vi "TagSync.vi"() -> ()   [LabVIEW 2015]
uses:
  <vilib>/Utility/error.llb/DialogType.ctl
  <resource>/objmgr/daqmx.rc
  <vilib>/DAQmx/configure/timing.llb/DAQmx Timing (Sample Clock).vi
  <vilib>/DAQmx/create/channels.llb/DAQmx Create Channel (DO-Digital Output).vi
  <vilib>/DAQmx/write.llb/DAQmx Write (Digital Wfm 1Chan NSamp).vi
panel:
  in  "Sync Tagging":T1(tab)
  out "Minimum tagging period (pws)":u32=87
  out "Total tag data length (pws)":i32=86
  in  "Tagging Period (pws)":u32=155
  in  "Calculate recommended tag settings":bool
  in  "Validate tag settings":bool
  in  "Tag Marker Duration (pws)":i32=10
  in  "Requested Pulse Width (ms)":dbl=10.0
  out "Actual pulse width (ms)":dbl=-1.0
  in  "Sync Tag Output Line":tag
  in  "Sample Clock Source":tag
  out "Current tag period":digitalwaveform(graph)
  out "Current tag ID":u32=1
  in  "Enable monitoring":bool
  in  "Min extra tag separation (pws)":u32=1
  in  "Minimum tags per file":u32=3
  in  "Minimum samples per pulse":dbl=10.0 format="%#_13g"
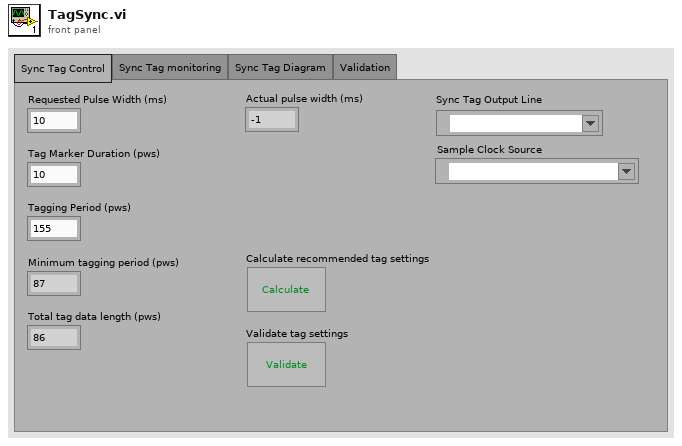
[diagram p1: front panel]
types:
  T1 = enum32{"Sync Tag Control", "Sync Tag monitoring", "Sync Tag Diagram", "Validation"}
  T2 = typedef "DialogType.ctl" = u16
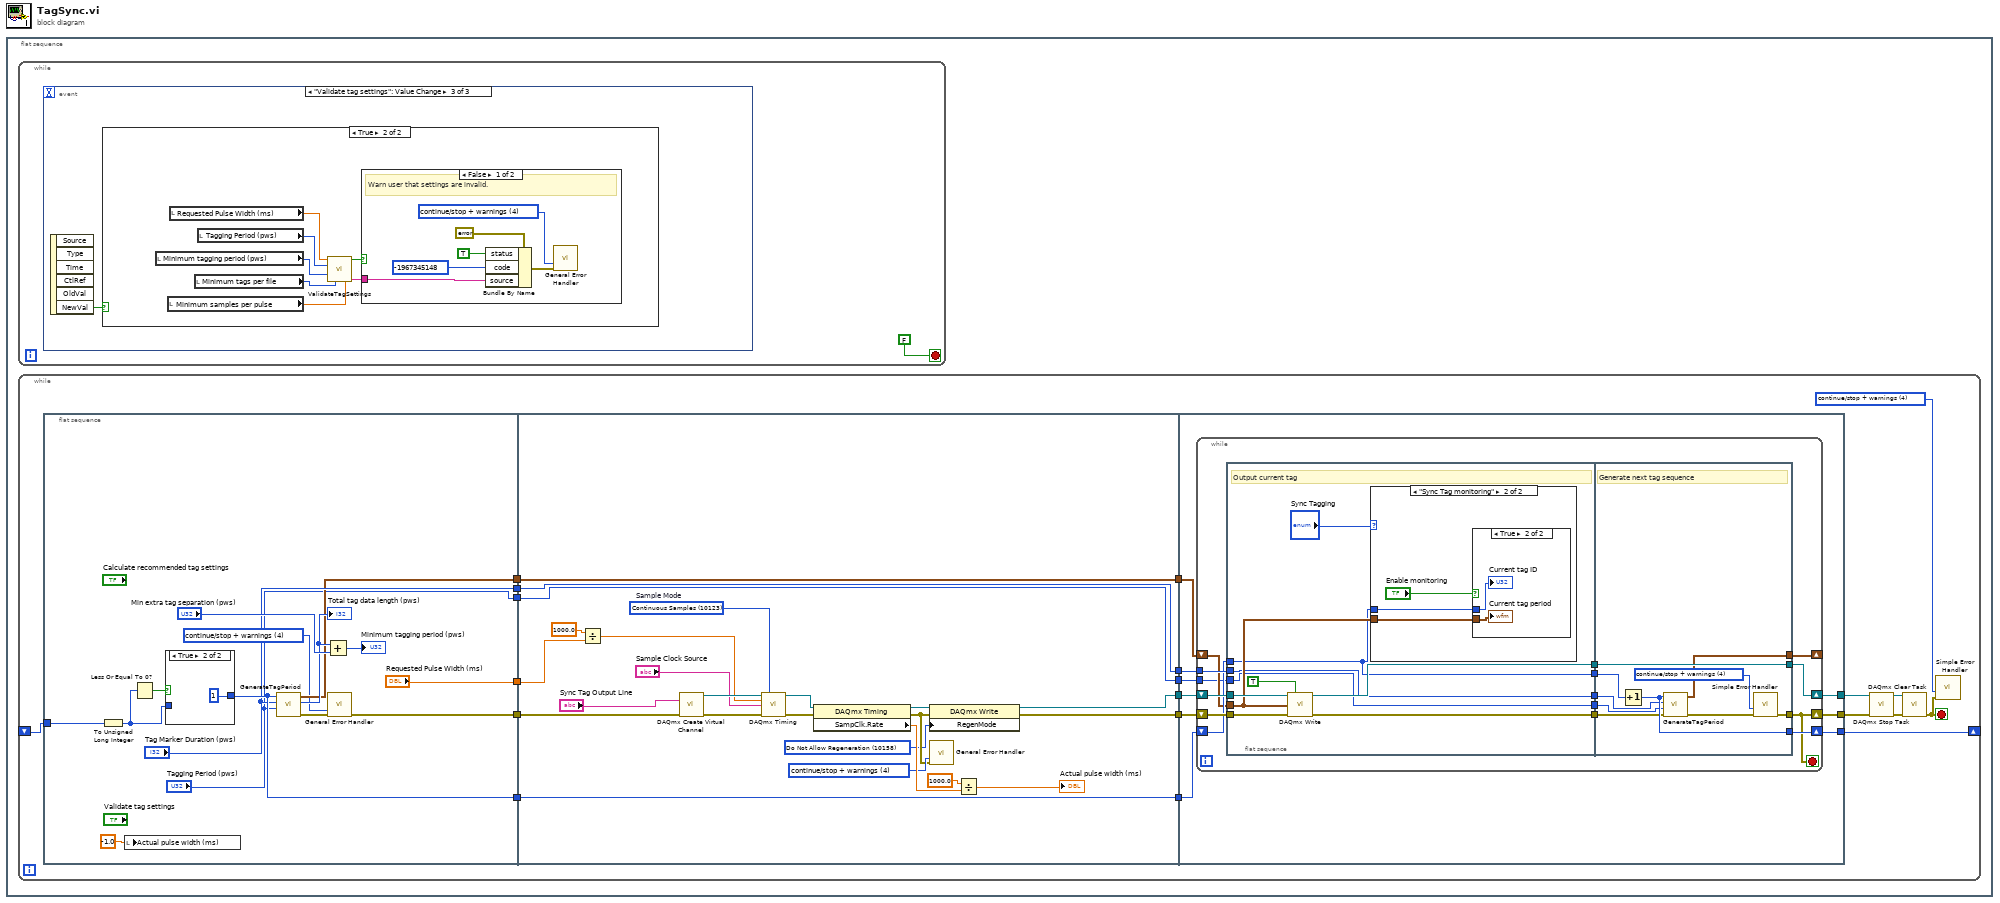
[diagram p0: block diagram]
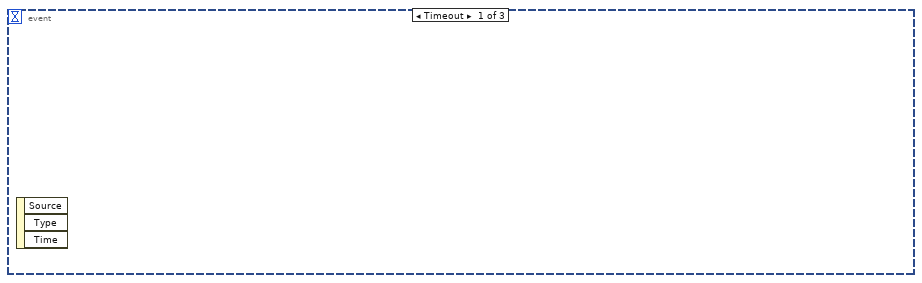
[diagram p5: hidden frame]
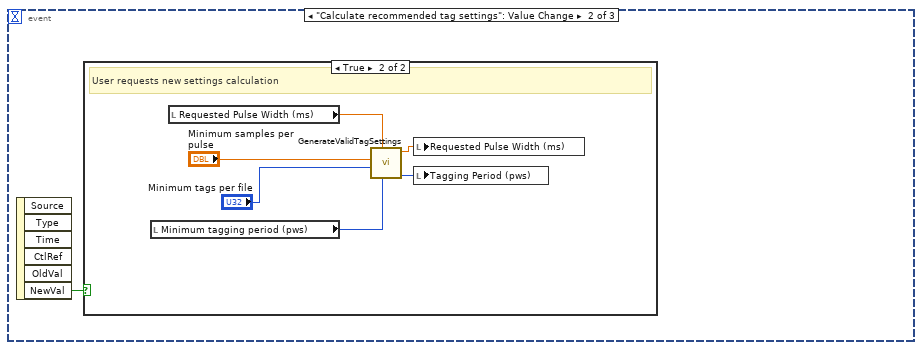
[diagram p6: hidden frame]
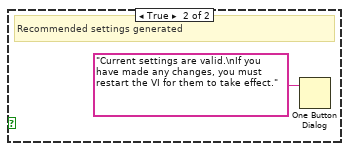
[diagram p9: hidden frame]
diagram:
  n1 = flat-sequence {
    frame #0 {
      n2 = while {
        stop <- FALSE stop-if-true
        n3 = event shown="[2] \"Validate tag settings\": Value Change" {
          selector: _ -> [_ _ _]
          dyn-events: _ -> [_ _ _]
          timeout: _ -> [_ _ _]
          event Timeout {
            n4 = event-data() -> ()  [unwired: 1 in, 3 out]
          }
          event "Calculate recommended tag settings": Value Change {
            n5 = event-data() -> ("NewVal"=w112:bool)  [unwired: 1 in, 5 out]
            n6 = case shown="True" w112 {
              frame False {
              }
              frame True {
                # "User requests new settings calculation"
                n7 = local read "Minimum tagging period (pws)"() -> (w118:u32)
                n8 = local read "Requested Pulse Width (ms)"() -> (w115:dbl)
                n9 = call "GenerateValidTagSettings.vi"("Minimum tagging period (pws)"=w118, "PulseWidth (ms)"=w115, "Minimum tags per file"="Minimum tags per file", "Minimum samples per pulse"="Minimum samples per pulse") -> ("TaggingPeriod (pws)"=w114:u32, "Valid Pulse Width (ms)"=w116:dbl)  [unwired: 6 in]
                n10 = local write "Requested Pulse Width (ms)"(w116) -> ()
                n11 = local write "Tagging Period (pws)"(w114) -> ()
              }
            }
          }
          event "Validate tag settings": Value Change {
            n12 = event-data() -> ("NewVal"=w119:bool)  [unwired: 1 in, 5 out]
            n13 = case shown="True" w119 {
              frame False {
              }
              frame True {
                n14 = local read "Minimum tagging period (pws)"() -> (w126:u32)
                n15 = local read "Minimum samples per pulse"() -> (w125:dbl)
                n16 = local read "Requested Pulse Width (ms)"() -> (w122:dbl)
                n17 = local read "Minimum tags per file"() -> (w124:u32)
                n18 = local read "Tagging Period (pws)"() -> (w123:u32)
                n19 = call "ValidateTagSettings.vi"("PulseWidth (ms)"=w122, "TaggingPeriod (pws)"=w123, "Minimum tagging period (pws)"=w126, "Minimum tags per file"=w124, "Minimum samples per pulse"=w125) -> ("Valid"=w121:bool, "Info"=w120:string)  [unwired: 9 in]
                n20 = case shown="False" w121 {
                  tunnel: w120 -> [w127 _]
                  frame False {
                    w132 = T2 4 items=["no dialog", "OK message", "continue or stop message", "OK message + warnings", "continue/stop + warnings"] ("type of dialog (OK msg:1)")
                    # "Warn user that settings are invalid."
                    n21 = Bundle By Name(cluster=errorcluster {"status"=FALSE, "code"=0, "source"=""} ("error in (no error)"), "status"=TRUE, "code"=-1967345148, "source"=w127) -> (w131:errorcluster)
                    n22 = call <vilib>:"General Error Handler.vi"("type of dialog (OK msg:1)"=w132, "error in (no error)"=w131) -> ()  [unwired: 9 in, 5 out]
                  }
                  frame True {
                    # "Recommended settings generated"
                    n23 = One Button Dialog(message="Current settings are valid.\nIf you have made any changes, you must restart the VI for them to take effect.") -> ()  [unwired: 1 in, 1 out]
                  }
                }
              }
            }
          }
        }
      }
      n24 = while {
        shift-right: [w9] -> _
        shift-left: _ -> [w10]
        stop <- w4 stop-if-true
        w13 = T2 4 items=["no dialog", "OK message", "continue or stop message", "OK message + warnings", "continue/stop + warnings"] ("type of dialog (OK msg:1)")
        n25 = flat-sequence {
          tunnel: ["Tag Marker Duration (pws)"] -> w8
          tunnel: [w28] -> w7
          tunnel: [w25] -> w6
          tunnel: ["Requested Pulse Width (ms)"] -> w5
          tunnel: w10 -> [w31]
          tunnel: [w22] -> w3
          tunnel: ["Tagging Period (pws)"] -> w1
          tunnel: [w41] -> w20
          tunnel: [w42] -> w19
          tunnel: [w56] -> w18
          tunnel: w8 -> [w56]
          tunnel: [w55] -> w17
          tunnel: w7 -> [w55]
          tunnel: [w54] -> w16
          tunnel: w6 -> [w54]
          tunnel: w5 -> [w45]
          tunnel: w3 -> [w39]
          tunnel: [w38] -> w2
          tunnel: w1 -> [w38]
          tunnel: [w70] -> w12
          tunnel: [w69] -> w11
          tunnel: w20 -> [w68]
          tunnel: w19 -> [w67]
          tunnel: w18 -> [w66]
          tunnel: w17 -> [w65]
          tunnel: w16 -> [w64]
          tunnel: [w63] -> w9
          tunnel: w2 -> [w62]
          frame #0 {
            w24 = T2 4 items=["no dialog", "OK message", "continue or stop message", "OK message + warnings", "continue/stop + warnings"] ("type of dialog (OK msg:1)")
            n26 = To Unsigned Long Integer(number=w31) -> (unsigned 32bit integer=w29:u32)
            n27 = local write "Actual pulse width (ms)"(-1.0 ("Actual pulse width")) -> ()
            n28 = Less Or Equal To 0?(x=w29) -> (x <= 0?=w30:bool)
            n29 = case shown="True" w30 {
              tunnel: w29 -> [w36 _]
              tunnel: [w36 u32 1] -> w28
              frame False {
              }
              frame True {
              }
            }
            n30 = call "GenerateTagPeriod.vi"("TaggingPeriod (pws)"="Tagging Period (pws)", "TagMarkerDuration (pws)"="Tag Marker Duration (pws)", "Tag num"=w28) -> ("Error Out"=w23:errorcluster, "TagDataLength (pws)"=w26:i32, "TagPeriodData"=w25:digitalwaveform)  [unwired: 6 in]
            "Total tag data length (pws)" <- w26
            n31 = Add(x=w26, y="Min extra tag separation (pws)") -> (x+y=→"Minimum tagging period (pws)":u32)
            n32 = call <vilib>:"General Error Handler.vi"("type of dialog (OK msg:1)"=w24, "error in (no error)"=w23) -> ("error out"=w22:errorcluster)  [unwired: 9 in, 4 out]
          }
          frame #1 {
            w40 = 10158 items=["Allow Regeneration"=10097, "Do Not Allow Regeneration"=10158] ("RegenMode")
            w46 = T2 4 items=["no dialog", "OK message", "continue or stop message", "OK message + warnings", "continue/stop + warnings"] ("type of dialog (OK msg:1)")
            w57 = 10123 items=["Finite Samples"=10178, "Continuous Samples"=10123, "Hardware Timed Single Point"=12522]  # Sample Mode
            n33 = Divide(x=1000.0 ("y"), y=w45) -> (x/y=w52:dbl)
            n34 = call-poly <vilib>:"DAQmx Create Virtual Channel.vi"("lines"="Sync Tag Output Line", "error in"=w39) -> ("task out"=w58:refnum<k21>, "error out"=w59:errorcluster)  [unwired: 12 in]
            n35 = call-poly <vilib>:"DAQmx Timing.vi"("task/channels in"=w58, "sample mode"=w57, "rate"=w52, "source"="Sample Clock Source", "error in"=w59) -> ("task out"=w60:refnum<k21>, "error out"=w61:errorcluster)  [unwired: 9 in]
            n36 = property class="DAQmx Timing"(reference=w60, error in=w61) -> (reference out=w43:refnum<k21>, error out=w44:errorcluster, "SampClk.Rate"=w51:dbl)
            n37 = property class="DAQmx Write"(reference=w43, error in=w44, "RegenMode"=w40) -> (reference out=w42:refnum<k21>, error out=w41:errorcluster)
            n38 = call <vilib>:"General Error Handler.vi"("type of dialog (OK msg:1)"=w46, "error in (no error)"=w44) -> ()  [unwired: 9 in, 5 out]
            n39 = Divide(x=1000.0 ("y"), y=w51) -> (x/y=→"Actual pulse width (ms)":dbl)
          }
          frame #2 {
            n40 = while {
              shift-right: [w83] -> w70
              shift-left: w67 -> [w85]
              shift-right: [w71] -> w69
              shift-left: w68 -> [w84]
              tunnel: w66 -> [w82]
              shift-right: [w80] -> w63
              shift-left: w65 -> [w81]
              shift-right: [w72] -> _
              shift-left: w64 -> [w79]
              tunnel: w62 -> [w74]
              stop <- w71 stop-if-true
              n41 = flat-sequence {
                tunnel: [w90] -> w78
                tunnel: [w92] -> w77
                tunnel: [w93] -> w76
                tunnel: [w88] -> w75
                tunnel: w85 -> [w95]
                tunnel: w84 -> [w94]
                tunnel: w82 -> [w90]
                tunnel: w81 -> [w88]
                tunnel: w79 -> [w91]
                tunnel: w74 -> [w86]
                tunnel: [w86] -> w73
                tunnel: w78 -> [w106]
                tunnel: w77 -> [w104]
                tunnel: w76 -> [w110]
                tunnel: [w107] -> w80
                tunnel: [w110] -> w83
                tunnel: w75 -> [w108]
                tunnel: w73 -> [w105]
                tunnel: [w102] -> w71
                tunnel: [w101] -> w72
                frame #0 {
                  # "Output current tag"
                  n42 = call-poly <vilib>:"DAQmx Write.vi"("task/channels in"=w95, "auto start"=TRUE, "data"=w91, "error in"=w94) -> ("task out"=w93:refnum<k21>, "error out"=w92:errorcluster)  [unwired: 9 in, 1 out]
                  n43 = case shown="\"Sync Tag monitoring\"" "Sync Tagging" {
                    tunnel: w91 -> [_ w98]
                    tunnel: w88 -> [_ w97]
                    frame "Sync Tag Control", Default {
                    }
                    frame "Sync Tag monitoring" {
                      n44 = case shown="True" "Enable monitoring" {
                        tunnel: w98 -> [_ w100]
                        tunnel: w97 -> [_ w99]
                        frame False {
                        }
                        frame True {
                          "Current tag period" <- w100
                          "Current tag ID" <- w99
                        }
                      }
                    }
                  }
                }
                frame #1 {
                  w109 = T2 4 items=["no dialog", "OK message", "continue or stop message", "OK message + warnings", "continue/stop + warnings"] ("type of dialog (OK msg:1)")
                  # "Generate next tag sequence"
                  n45 = Increment(x=w108) -> (x+1=w107:u32)
                  n46 = call "GenerateTagPeriod.vi"("Error in"=w104, "TaggingPeriod (pws)"=w105, "TagMarkerDuration (pws)"=w106, "Tag num"=w107) -> ("Error Out"=w103:errorcluster, "TagPeriodData"=w101:digitalwaveform)  [unwired: 5 in, 1 out]
                  n47 = call <vilib>:"Simple Error Handler.vi"("type of dialog (OK msg:1)"=w109, "error in (no error)"=w103) -> ("error out"=w102:errorcluster)  [unwired: 3 in, 4 out]
                }
              }
            }
          }
        }
        n48 = call <vilib>:"DAQmx Stop Task.vi"("task/channels in"=w12, "error in"=w11) -> ("task out"=w15:refnum<k21>, "error out"=w14:errorcluster)  [unwired: 12 in]
        n49 = call <vilib>:"DAQmx Clear Task.vi"("task in"=w15, "error in"=w14) -> ("error out"=w4:errorcluster)  [unwired: 13 in]
        n50 = call <vilib>:"Simple Error Handler.vi"("type of dialog (OK msg:1)"=w13, "error in (no error)"=w4) -> ()  [unwired: 3 in, 5 out]
      }
    }
  }
